vi "GetSelectIndex.vi"(10 "Coords":T1, 11 "Array in":refnum<vi>) -> (3 "Index":cluster{"Row":i32, "Coloumn":i32})   [LabVIEW 2018]
uses:
  <vilib>/Utility/miscctls.llb/LVPoint32TypeDef.ctl
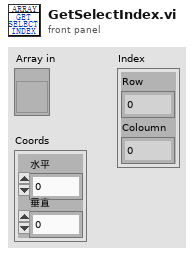
[diagram p1: front panel]
types:
  T1 = typedef "LVPoint32TypeDef.ctl" = cluster{"Horizontal":i32, "Vertical":i32}
  T2 = typedef "LVPositionTypeDef.ctl" = cluster{"Left":i32, "Top":i32}
  T3 = typedef "LVBoundsTypeDef.ctl" = cluster{"Width":u32, "Height":u32}
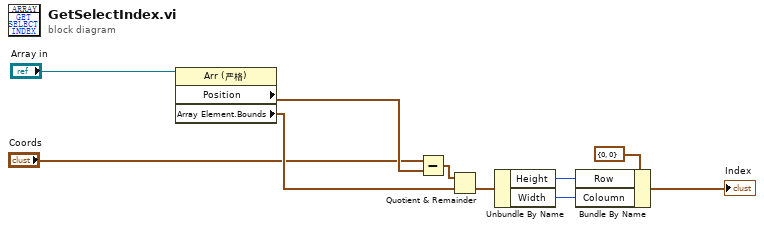
[diagram p0: block diagram]
diagram:
  n1 = property class="Arr (严格)"(reference="Array in") -> ("Position"=w3:T2, "Array Element.Bounds"=w5:T3)  [unwired: 1 in, 2 out]
  n2 = Subtract(x="Coords", y=w3) -> (x-y=w4:T1)
  n3 = Quotient & Remainder(x=w4, y=w5) -> (floor(x/y)=w7:T3)  [unwired: 1 out]
  n4 = Unbundle By Name(w7) -> ("Height"=w9:u32, "Width"=w10:u32)
  n5 = Bundle By Name(cluster=cluster{"Row":i32, "Coloumn":i32} {"Row"=0, "Coloumn"=0}, "Row"=w9, "Coloumn"=w10) -> (→"Index":cluster{"Row":i32, "Coloumn":i32})
